vi "Initialize From Settings.vi"(8 "error in":errorcluster, 10 "settings":cluster{"key":string, "value":string}[](array[cluster]), 11 "RDMA Rx Transfer Configuration in":refnum<class "RDMA Transfer Rx Configuration.lvclass">=refnum) -> (0 "error out":errorcluster, 3 "RDMA Rx Transfer Configuration out":refnum<class "RDMA Transfer Rx Configuration.lvclass">)   [LabVIEW 2020, in "RDMA.lvlib" / "RDMA Transfer Rx Configuration.lvclass"]
uses:
  RDMA Transfer Rx Configuration.lvclass
  Rx Transfer Settings.ctl
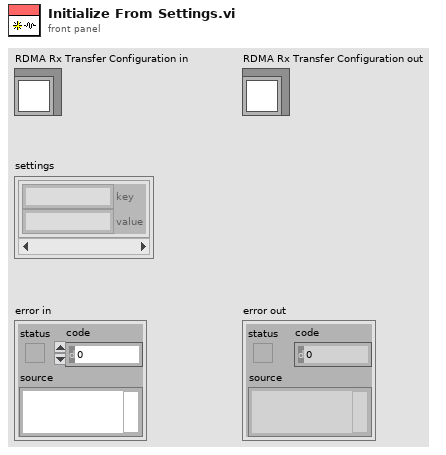
[diagram p1: front panel]
types:
  T1 = typedef "RDMA.lvlib/RDMA Transfer Rx Configuration.lvclass/Rx Transfer Settings.ctl" = cluster{"local address":u32, "local port":u16}
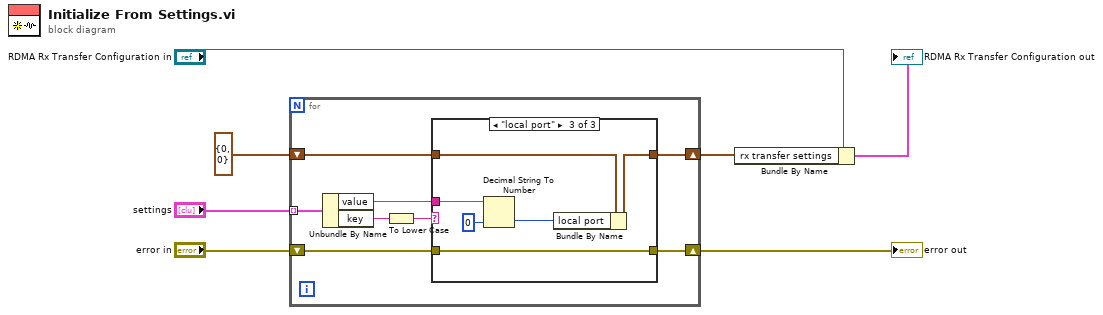
[diagram p0: block diagram]
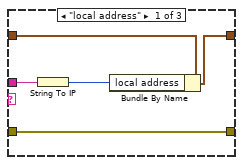
[diagram p2: hidden frame]
diagram:
  n1 = for {
    shift-right: [w10] -> w1
    shift-left: "error in" -> [w14]
    shift-right: [w12] -> w5
    shift-left: T1 {"local address"=0, "local port"=0} ("rx transfer settings") -> [w13]
    tunnel: "settings" -> [w15] mode=indexing
    n2 = Unbundle By Name(w15) -> ("value"=w9:string, "key"=w8:string)
    n3 = To Lower Case(string=w8) -> (all lower case string=w11:string)
    n4 = case shown="\"local port\"" w11 {
      tunnel: w14 -> [w18 w21 w26]
      tunnel: w9 -> [w17 _ w25]
      tunnel: w13 -> [w20 w22 w28]
      tunnel: [w19 w22 w27] -> w12
      tunnel: [w18 w21 w26] -> w10
      frame "local address" {
        n5 = String To IP(1:w17) -> (0:w16:u32)
        n6 = Bundle By Name(cluster=w20, "local address"=w16) -> (w19:T1)
      }
      frame Default {
        # "Unknown Setting:\nmay need to throw\nan error here"
      }
      frame "local port" {
        n7 = Decimal String To Number(string=w25, default (0L)=u16 0 ("default (0 I32)")) -> (number=w24:u16)  [unwired: 1 in, 1 out]
        n8 = Bundle By Name(cluster=w28, "local port"=w24) -> (w27:T1)
      }
    }
  }
  "error out" <- w1
  n9 = Bundle By Name(cluster="RDMA Rx Transfer Configuration in", "rx transfer settings"=w5) -> (→"RDMA Rx Transfer Configuration out":cluster{})
